vi "get_display_voltage_current_and_mode.vi"(8 "error in":errorcluster, 11 "VISA resource name":refnum<visa-resource-name>="COM1") -> (0 "error out":errorcluster, 3 "Response":string)   [LabVIEW 2020]
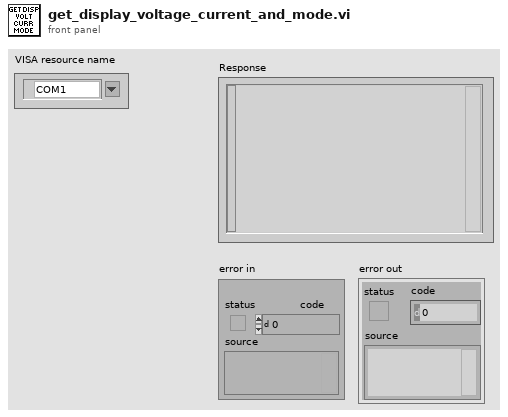
[diagram p1: front panel]
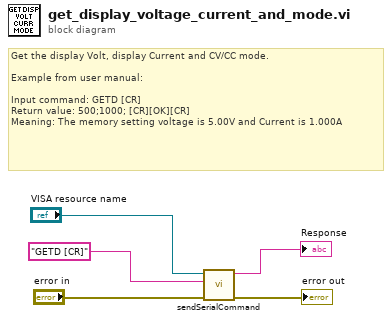
[diagram p0: block diagram]
diagram:
  # "Get the display Volt, display Current and CV/CC mode.\n\nExample from user manual:\n\nInput command: GETD [CR]\nReturn value: 500;1000; [CR][OK][CR]\nMeaning: The memory setting voltage is 5.00V and Current is 1.000A"
  n1 = call "sendSerialCommand.vi"("error in (no error)"="error in", "Command"="GETD [CR]", "VISA resource name"="VISA resource name") -> ("error out"=→"error out":errorcluster, "Response"=→"Response":string)  [unwired: 7 in]
